vi "Get Result.vi"(0 "reference in":refnum<class "Operation Context.lvclass">, 1 "x":dbl, 3 "y":dbl, 5 "error in (no error)":errorcluster, 6 "Operation.lvclass":refnum<class "Operation.lvclass">) -> (14 "reference out":refnum<class "Operation Context.lvclass">, 15 "result":dbl, 19 "error out":errorcluster)   [LabVIEW 2013, in "Operation Context.lvclass"]
uses:
  Operation Context.lvclass
  Operation_class/Operation.lvclass
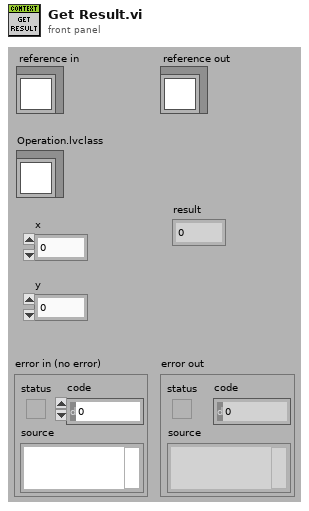
[diagram p1: front panel]
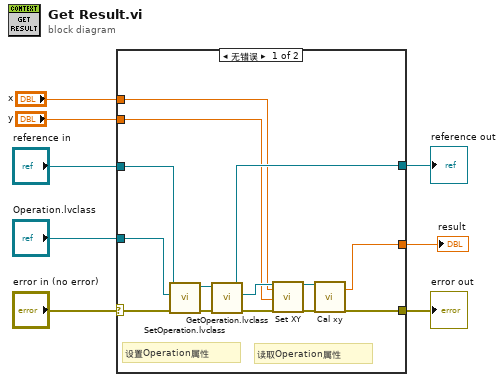
[diagram p0: block diagram]
diagram:
  n1 = case shown="无错误" "error in (no error)" {
    selector: "error in (no error)" -> [w18 w24]
    tunnel: [w14 w24] -> w7
    tunnel: [w13 w23] -> w5
    tunnel: "reference in" -> [w21 w23]
    tunnel: "Operation.lvclass" -> [w12 _]
    tunnel: "x" -> [w11 _]
    tunnel: "y" -> [w10 _]
    tunnel: [w9 _] -> w1
    frame No Error {
      # "读取Operation属性"
      # "设置Operation属性"
      n2 = call "SetOperation.lvclass.vi"("error in (no error)"=w18, "Operation.lvclass"=w12, "reference in"=w21) -> ("error out"=w20:errorcluster, "reference out"=w22:refnum<class "Operation Context.lvclass">)  [unwired: 7 in]
      n3 = call "GetOperation.lvclass.vi"("error in (no error)"=w20, "reference in"=w22) -> ("error out"=w17:errorcluster, "Operation.lvclass"=w19:refnum<class "Operation.lvclass">, "reference out"=w13:refnum<class "Operation Context.lvclass">)  [unwired: 7 in]
      n4 = call "Set XY.vi"("reference in"=w19, "x"=w11, "y"=w10, "error in (no error)"=w17) -> ("reference out"=w16:refnum<class "Operation.lvclass">, "error out"=w15:errorcluster)  [unwired: 14 in]
      n5 = call-dynamic "Cal xy.vi"("reference in"=w16, "error in (no error)"=w15) -> ("result"=w9:dbl, "error out"=w14:errorcluster)  [unwired: 15 in, 1 out]
    }
    frame Error {
    }
  }
  "error out" <- w7
  "reference out" <- w5
  "result" <- w1
